vi "LecturaCorreccions.vi"(8 "error in (no error)":errorcluster, 10 "String":string, 11 "Cluster in":refnum<vi>) -> (0 "error out":errorcluster, 2 "CorreccioNegativa":T1, 3 "CorreccioPositiva":T1)   [LabVIEW 2017]
uses:
  <vilib>/registry/registry.llb/Registry RtKey.ctl
  <vilib>/registry/registry.llb/Read Registry Value Simple STR.vi
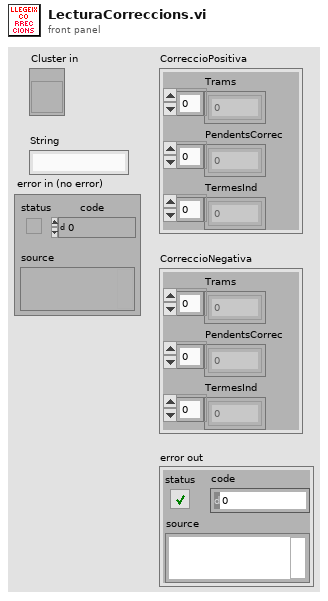
[diagram p1: front panel]
types:
  T1 = cluster{"Trams":dbl[], "PendentsCorrec":dbl[], "TermesInd":dbl[]}
  T2 = typedef "Registry RtKey.ctl" = enum32{"HKEY_CLASSES_ROOT", "HKEY_CURRENT_USER", "HKEY_LOCAL_MACHINE", "HKEY_USERS", "HKEY_PERFORMANCE_DATA", "HKEY_CURRENT_CONFIG", "HKEY_DYN_DATA"}
  T3 = typedef "Registry refnum.ctl" = refnum<k1>
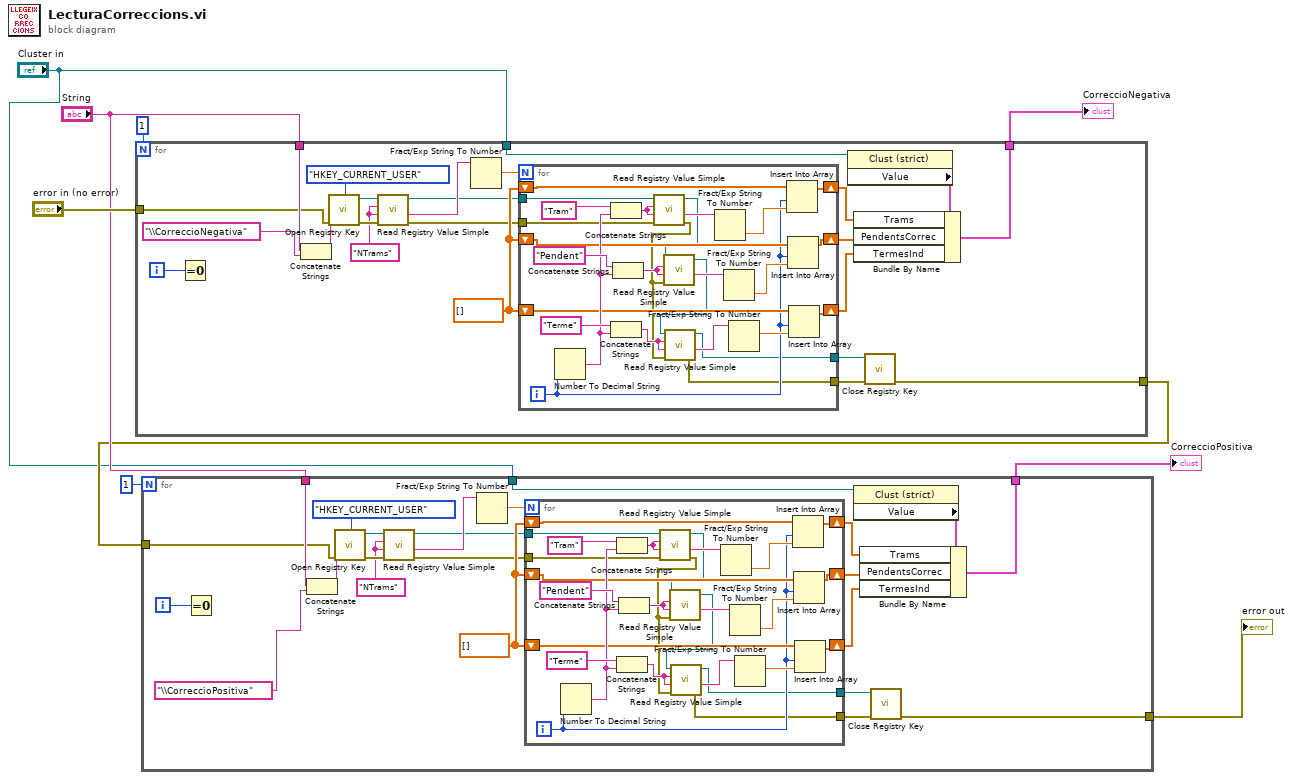
[diagram p0: block diagram]
diagram:
  n1 = for {
    N: 1 -> [_]
    tunnel: "String" -> [w27]
    tunnel: [w15] -> w4
    tunnel: [w10] -> w9
    tunnel: "Cluster in" -> [w13]
    tunnel: "error in (no error)" -> [w12]
    i -> [w20]
    w23 = "NTrams" ("value")
    w21 = dbl[] [] ("Trams")
    n2 = Equal To 0?(x=w20) -> ()  [unwired: 1 out]
    n3 = Concatenate Strings(w27, "\\CorreccioNegativa" ("subkey")) -> (w26:string)
    n4 = call <vilib>:"Open Registry Key.vi"("error in (no error)"=w12, "subkey"=w26, "root key (HKEY_LOCAL_MACHINE)"=Registry_RtKey."HKEY_CURRENT_USER") -> ("error out"=w24:errorcluster, "refnum out"=w25:T3)  [unwired: 7 in]
    n5 = call-poly <vilib>:"Read Registry Value Simple.vi"("error in (no error)"=w24, "default data"=w23, "value"=w23, "refnum"=w25) -> ("error out"=w18:errorcluster, "String/Binary data"=w22:string, "refnum out"=w19:T3)  [unwired: 2 in, 1 out]
    n6 = Fract/Exp String To Number(string=w22) -> (number=w32:dbl)  [unwired: 3 in, 1 out]
    n7 = for {
      N: w32 -> [_]
      shift-right: [w49] -> w31
      shift-left: w21 -> [w50]
      shift-right: [w47] -> w30
      shift-left: w21 -> [w46]
      shift-right: [w43] -> w29
      shift-left: w21 -> [w44]
      tunnel: w19 -> [w40]
      tunnel: w18 -> [w39]
      tunnel: [w34] -> w17
      tunnel: [w33] -> w16
      i -> [w41]
      n8 = Number To Decimal String(number=w41) -> (decimal integer string=w53:string)  [unwired: 1 in]
      n9 = Concatenate Strings("Tram" ("value"), w53) -> (w58:string)
      n10 = Concatenate Strings("Terme" ("value"), w53) -> (w52:string)
      n11 = Concatenate Strings("Pendent" ("value"), w53) -> (w37:string)
      n12 = call-poly <vilib>:"Read Registry Value Simple.vi"("error in (no error)"=w39, "default data"=w58, "value"=w58, "refnum"=w40) -> ("error out"=w35:errorcluster, "String/Binary data"=w57:string, "refnum out"=w38:T3)  [unwired: 2 in, 1 out]
      n13 = call-poly <vilib>:"Read Registry Value Simple.vi"("error in (no error)"=w35, "default data"=w37, "value"=w37, "refnum"=w38) -> ("String/Binary data"=w55:string, "refnum out"=w36:T3)  [unwired: 2 in, 2 out]
      n14 = call-poly <vilib>:"Read Registry Value Simple.vi"("error in (no error)"=w35, "default data"=w52, "value"=w52, "refnum"=w36) -> ("error out"=w34:errorcluster, "String/Binary data"=w51:string, "refnum out"=w33:T3)  [unwired: 2 in, 1 out]
      n15 = Fract/Exp String To Number(string=w57) -> (number=w48:dbl)  [unwired: 3 in, 1 out]
      n16 = Fract/Exp String To Number(string=w55) -> (number=w45:dbl)  [unwired: 3 in, 1 out]
      n17 = Fract/Exp String To Number(string=w51) -> (number=w42:dbl)  [unwired: 3 in, 1 out]
      n18 = Insert Into Array(array=w50, index=w41, new element=w48) -> (w49:dbl[])
      n19 = Insert Into Array(array=w46, index=w41, new element=w45) -> (w47:dbl[])
      n20 = Insert Into Array(array=w44, index=w41, new element=w42) -> (w43:dbl[])
    }
    n21 = property on="Property Node" class="Clust (strict)"(reference=w13) -> ("Value"=w14:T1)  [unwired: 1 in, 2 out]
    n22 = Bundle By Name(cluster=w14, "Trams"=w31, "PendentsCorrec"=w30, "TermesInd"=w29) -> (w10:T1)
    n23 = call <vilib>:"Close Registry Key.vi"("error in (no error)"=w17, "refnum"=w16) -> ("error out"=w15:errorcluster)  [unwired: 5 in]
  }
  "CorreccioNegativa" <- w9
  n24 = for {
    N: 1 -> [_]
    tunnel: "String" -> [w77]
    tunnel: [w65] -> w3
    tunnel: [w60] -> w1
    tunnel: "Cluster in" -> [w63]
    tunnel: w4 -> [w62]
    i -> [w70]
    w73 = "NTrams" ("value")
    w71 = dbl[] [] ("Trams")
    n25 = Equal To 0?(x=w70) -> ()  [unwired: 1 out]
    n26 = Concatenate Strings(w77, "\\CorreccioPositiva" ("subkey")) -> (w76:string)
    n27 = call <vilib>:"Open Registry Key.vi"("error in (no error)"=w62, "subkey"=w76, "root key (HKEY_LOCAL_MACHINE)"=Registry_RtKey."HKEY_CURRENT_USER") -> ("error out"=w74:errorcluster, "refnum out"=w75:T3)  [unwired: 7 in]
    n28 = call-poly <vilib>:"Read Registry Value Simple.vi"("error in (no error)"=w74, "default data"=w73, "value"=w73, "refnum"=w75) -> ("error out"=w68:errorcluster, "String/Binary data"=w72:string, "refnum out"=w69:T3)  [unwired: 2 in, 1 out]
    n29 = Fract/Exp String To Number(string=w72) -> (number=w82:dbl)  [unwired: 3 in, 1 out]
    n30 = for {
      N: w82 -> [_]
      shift-right: [w99] -> w81
      shift-left: w71 -> [w100]
      shift-right: [w97] -> w80
      shift-left: w71 -> [w96]
      shift-right: [w93] -> w79
      shift-left: w71 -> [w94]
      tunnel: w69 -> [w90]
      tunnel: w68 -> [w89]
      tunnel: [w84] -> w67
      tunnel: [w83] -> w66
      i -> [w91]
      n31 = Number To Decimal String(number=w91) -> (decimal integer string=w103:string)  [unwired: 1 in]
      n32 = Concatenate Strings("Tram" ("value"), w103) -> (w108:string)
      n33 = Concatenate Strings("Terme" ("value"), w103) -> (w102:string)
      n34 = Concatenate Strings("Pendent" ("value"), w103) -> (w87:string)
      n35 = call-poly <vilib>:"Read Registry Value Simple.vi"("error in (no error)"=w89, "default data"=w108, "value"=w108, "refnum"=w90) -> ("error out"=w85:errorcluster, "String/Binary data"=w107:string, "refnum out"=w88:T3)  [unwired: 2 in, 1 out]
      n36 = call-poly <vilib>:"Read Registry Value Simple.vi"("error in (no error)"=w85, "default data"=w87, "value"=w87, "refnum"=w88) -> ("String/Binary data"=w105:string, "refnum out"=w86:T3)  [unwired: 2 in, 2 out]
      n37 = call-poly <vilib>:"Read Registry Value Simple.vi"("error in (no error)"=w85, "default data"=w102, "value"=w102, "refnum"=w86) -> ("error out"=w84:errorcluster, "String/Binary data"=w101:string, "refnum out"=w83:T3)  [unwired: 2 in, 1 out]
      n38 = Fract/Exp String To Number(string=w107) -> (number=w98:dbl)  [unwired: 3 in, 1 out]
      n39 = Fract/Exp String To Number(string=w105) -> (number=w95:dbl)  [unwired: 3 in, 1 out]
      n40 = Fract/Exp String To Number(string=w101) -> (number=w92:dbl)  [unwired: 3 in, 1 out]
      n41 = Insert Into Array(array=w100, index=w91, new element=w98) -> (w99:dbl[])
      n42 = Insert Into Array(array=w96, index=w91, new element=w95) -> (w97:dbl[])
      n43 = Insert Into Array(array=w94, index=w91, new element=w92) -> (w93:dbl[])
    }
    n44 = property on="Property Node" class="Clust (strict)"(reference=w63) -> ("Value"=w64:T1)  [unwired: 1 in, 2 out]
    n45 = Bundle By Name(cluster=w64, "Trams"=w81, "PendentsCorrec"=w80, "TermesInd"=w79) -> (w60:T1)
    n46 = call <vilib>:"Close Registry Key.vi"("error in (no error)"=w67, "refnum"=w66) -> ("error out"=w65:errorcluster)  [unwired: 5 in]
  }
  "CorreccioPositiva" <- w1
  "error out" <- w3
